vi "Autonomous Independent.vi"() -> ()   [LabVIEW 2012]
doc: "This VI is called when autonomous begins, and will automatically be terminated when autonomous ends. You can carry out timed or sensor driven robot movement independently without needing to return to the caller."
uses:
  <vilib>/Rock Robotics/WPI/Relay/WPI_RelayValue.ctl
  <vilib>/Rock Robotics/WPI/RobotDrive/WPI_RobotDriveGetSetRefNum.vi
  Robot Global Data.vi
panel:
  out "Shooter Up":bool
  out "Shooter Speed":T1(ring)
  out "Stop Drive":bool
  out "DT Output":enum16{"Off", "Up", "Down"}(ring)=enum."Down"
  out "DAD Up":bool
  out "DAD Output":T2
  out "Shift Low":bool
  out "Feeder Happy":bool
  out "Auton Done":bool
  out "Shooter Happy":bool
  out "Shoot!":bool
  out "Delay Switch":u32
  out "Seccond Switch":u32
  out "First Switch":u32
  # "Be sure to right-click and choose Data Operations>>Make Current Value default if you want to save the array values with the VI"
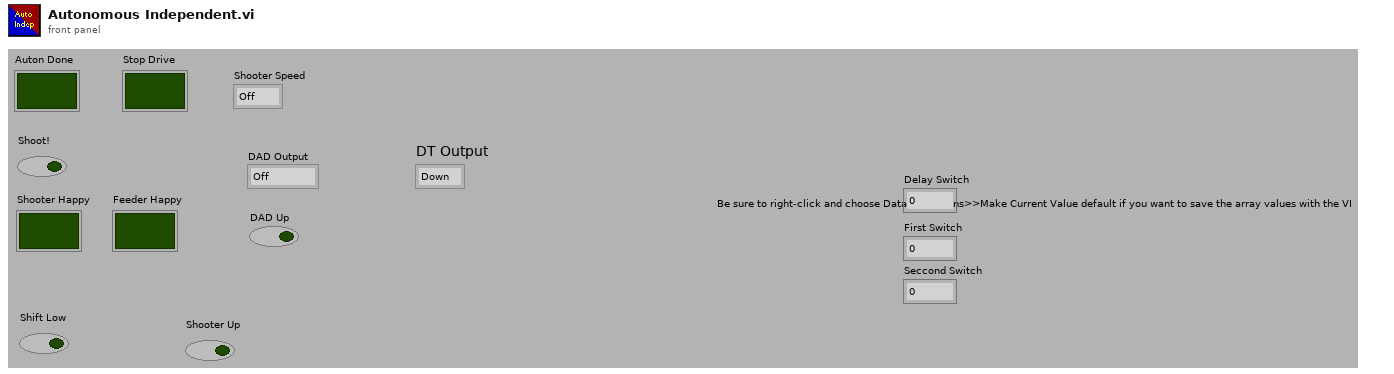
[diagram p1: front panel]
types:
  T1 = enum16{"Off", "Close Pyramid 3pt", "Far Pyramid 3pt", "Feeder Shot", "UD Far 3pt Shot"}
  T2 = typedef "WPI_RelayValue.ctl" = enum16{"Off", "On", "Forward", "Reverse"}
  T3 = enum16{"Off", "Close Pyramid 3pt", "Far Pyramid 3pt", "Feeder Shot"}
  T4 = typedef "WPI_RobotDriveDevRef.ctl" = cluster{"DevStatus":errorcluster, "Motors[]":T5[], "Square Inputs":bool, "Max Output":dbl, "Isochronous":bool}
  T5 = typedef "WPI_MotorControlDeviceRef.ctl" = cluster{"DeviceStatus":errorcluster, "Type":enum16{"PWM", "CAN"}, "PWM":cluster{"Digital Module":T6, "PWM Channel":T7, "DeadBand":T8}, "CAN":cluster{"Device Number":u8, "Control Mode":T9, "Semaphore":T10, "Max Vout":dbl}, "Invert":bool, "TransformRef":T11, "InvTransformRef":T11}
  T6 = typedef "FPGA_TypedefDigitalModule.ctl" = enum16{"Digital Module 1", "Digital Module 2"}
  T7 = typedef "FPGA_DIOPWMChannel.ctl" = enum8{"PWM 1", "PWM 2", "PWM 3", "PWM 4", "PWM 5", "PWM 6", "PWM 7", "PWM 8", "PWM 9", "PWM 10", "Invalid"}
  T8 = typedef "WPI_PWMDeadband.ctl" = cluster{"Name":string, "maxPositivePwm":i32, "minPositivePwm":i32, "centerPwm":i32, "maxNegativePwm":i32, "minNegativePwm":i32, "angularRange":u16}
  T9 = typedef "WPI_CANJaguar_ControlMode.ctl" = enum8{"Percent VBus", "Current", "Speed", "Position", "Voltage"}
  T10 = typedef "Semaphore RefNum" = refnum<k1>
  T11 = typedef "WPI_PWMTransform_ConPane.ctl" = refnum<vi>
  T12 = typedef "WPI_GyroDevRef.ctl" = cluster{"DevStatus":errorcluster, "Analog Module":T13, "Analog Channel":T14, "Offset":dbl, "Gain (VoltsPerDegree/Second)":dbl}
  T13 = typedef "FPGA_TypedefAnalogModule.ctl" = enum16{"Analog Module 1", "Analog Module 2"}
  T14 = typedef "FPGA_AIChannel.ctl" = enum8{"AI 1", "AI 2", "AI 3", "AI 4", "AI 5", "AI 6", "AI 7", "AI 8", "Invalid"}
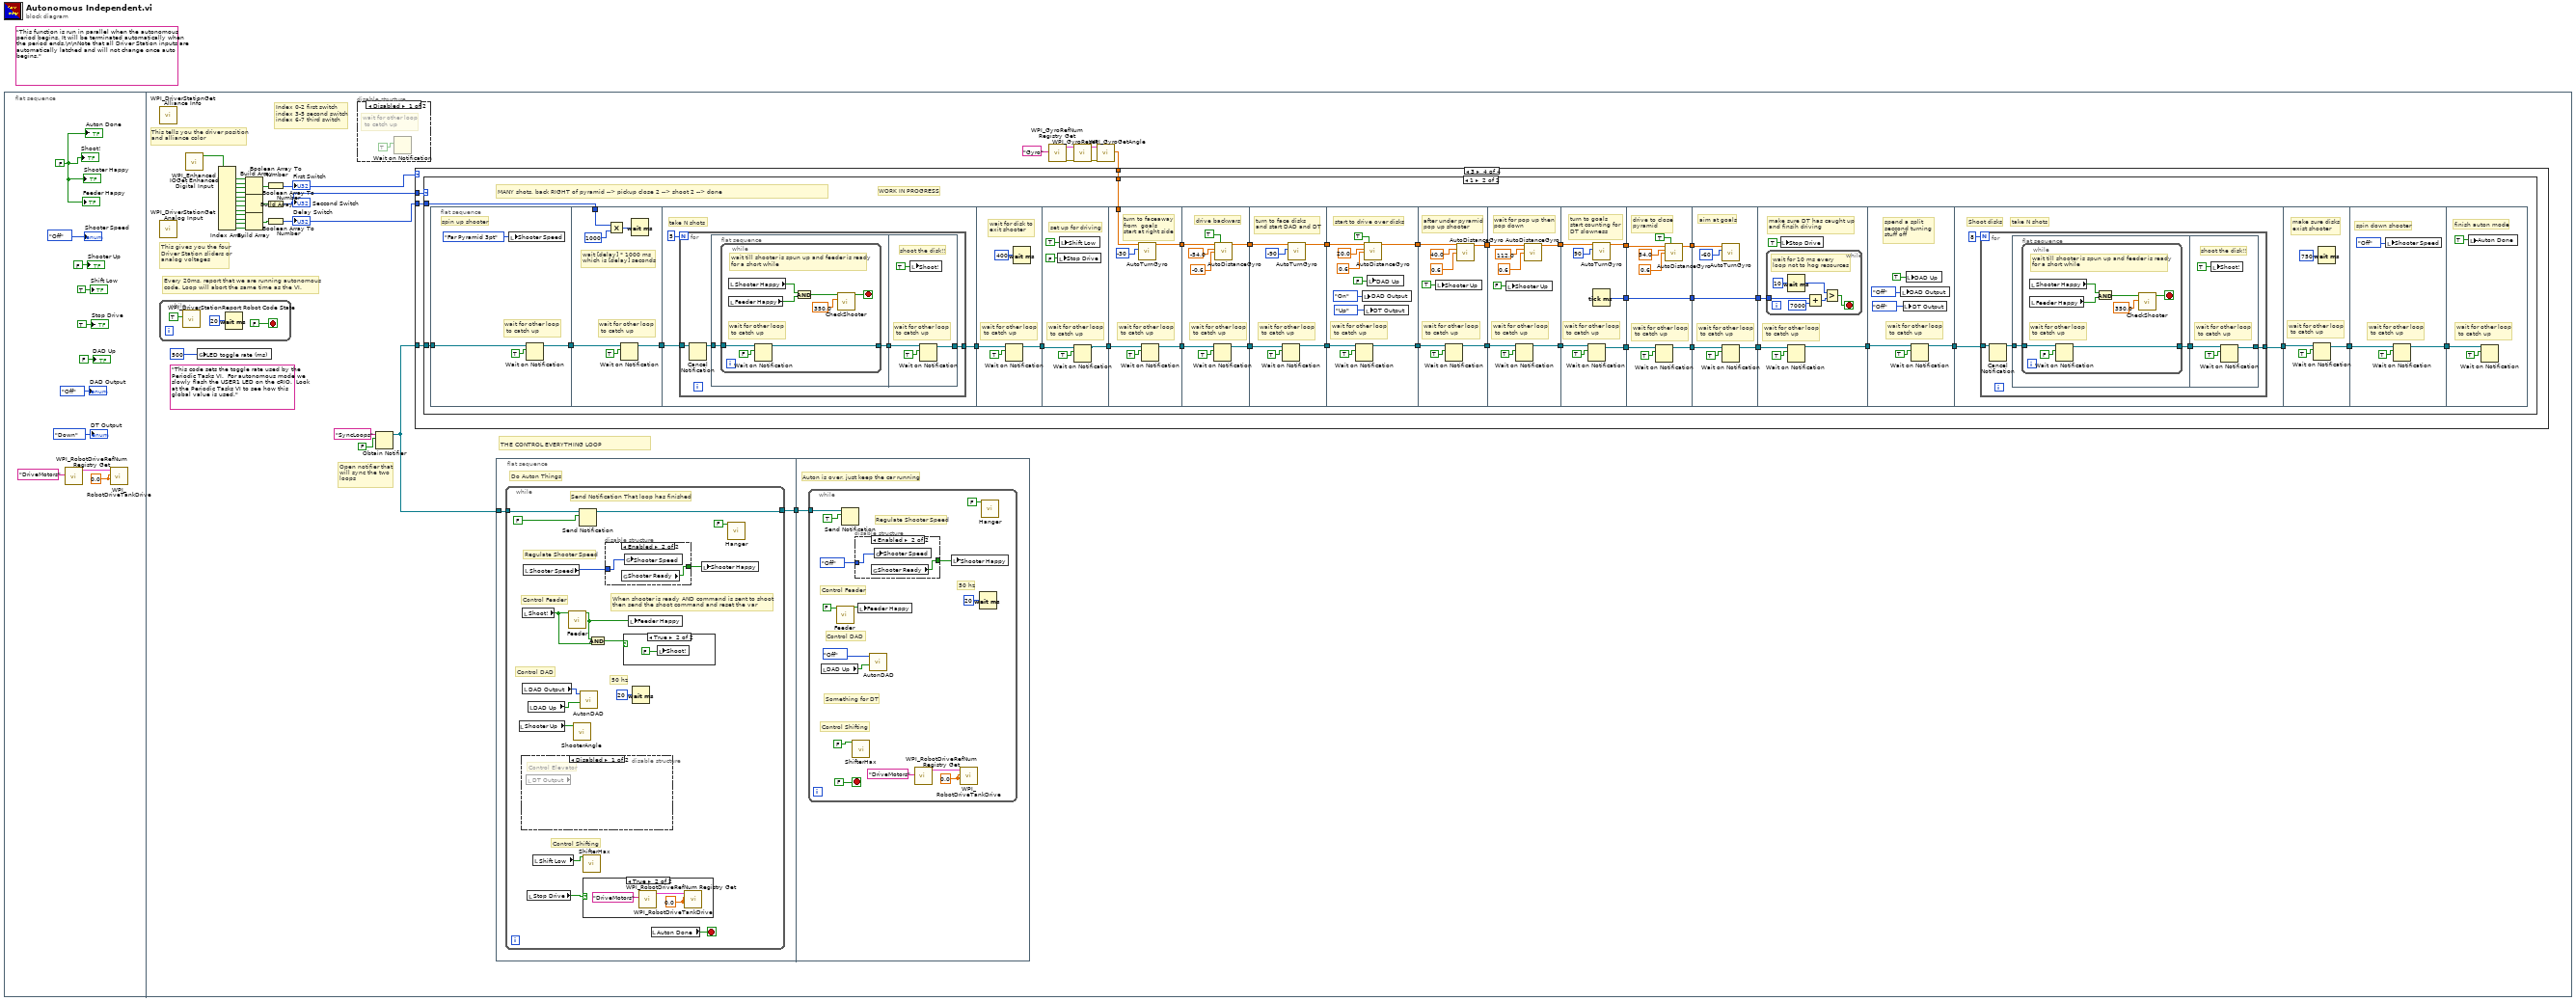
[diagram p0: block diagram]
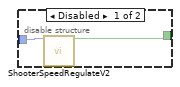
[diagram p3: hidden frame]
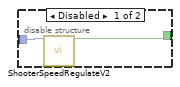
[diagram p7: hidden frame]
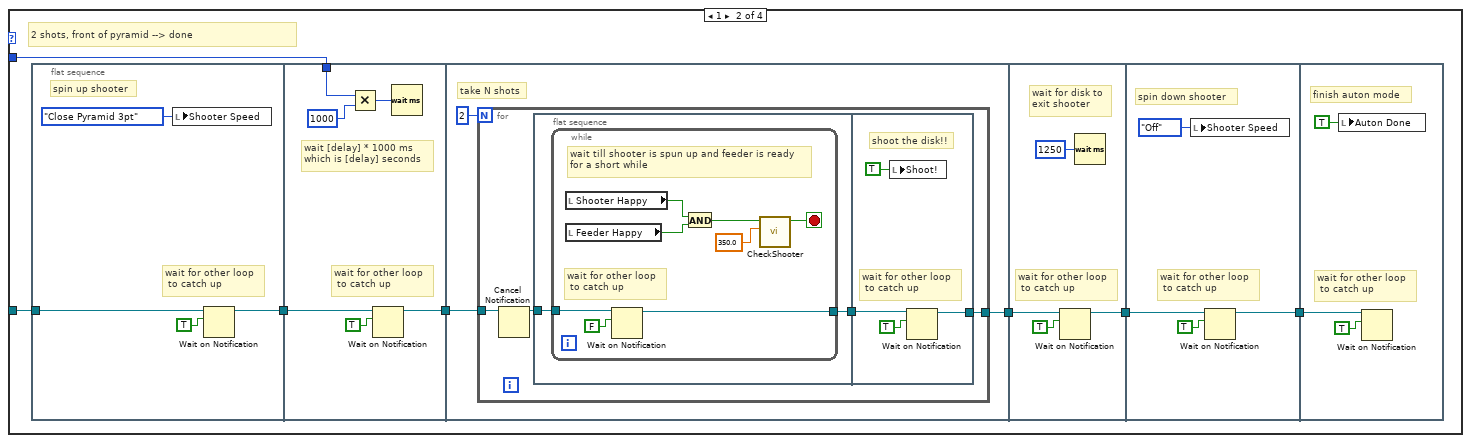
[diagram p10: hidden frame]
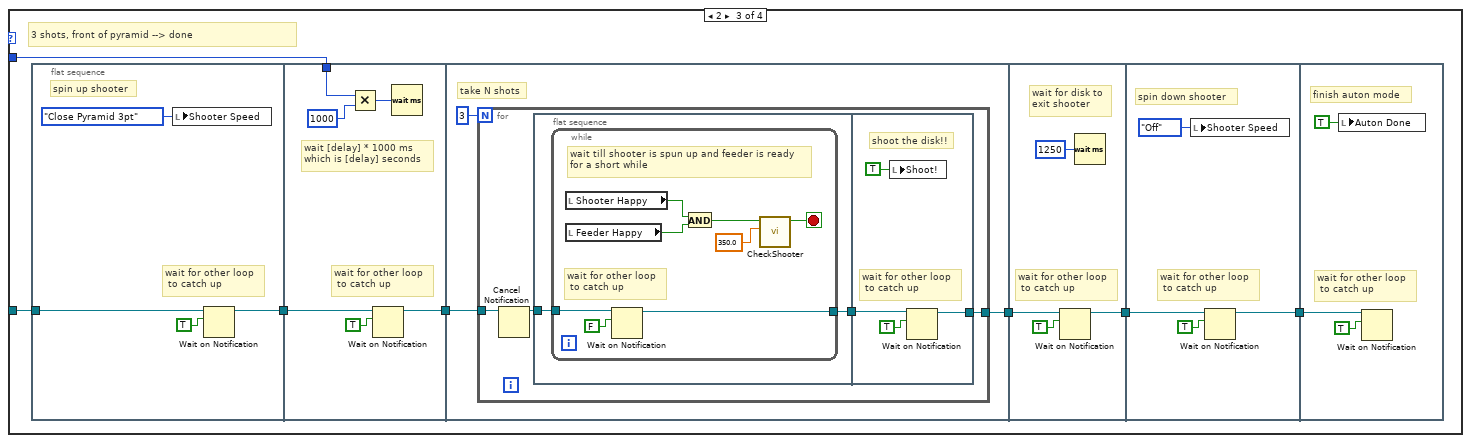
[diagram p11: hidden frame]
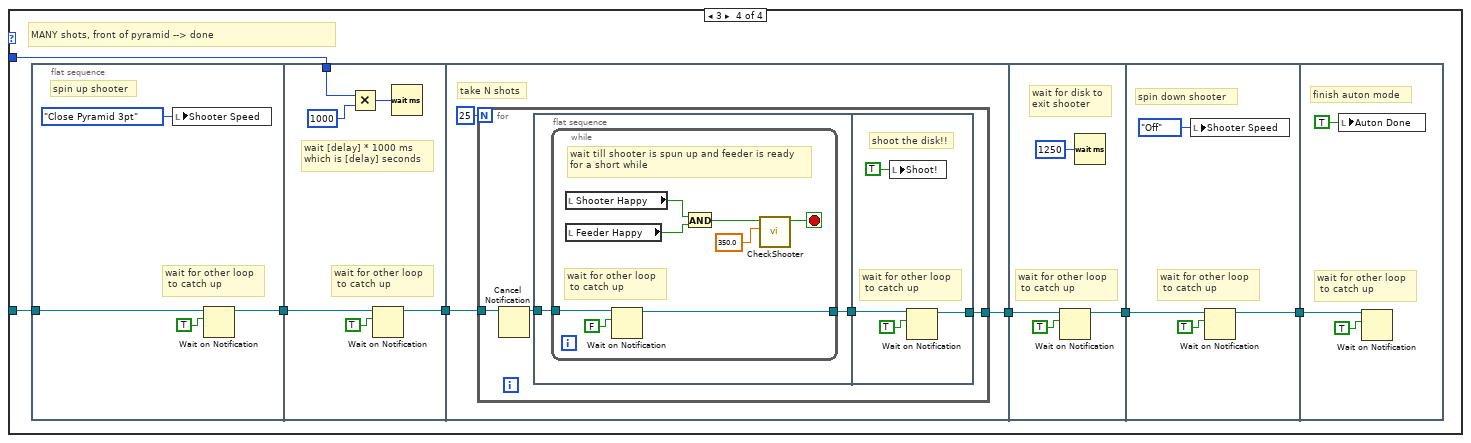
[diagram p12: hidden frame]
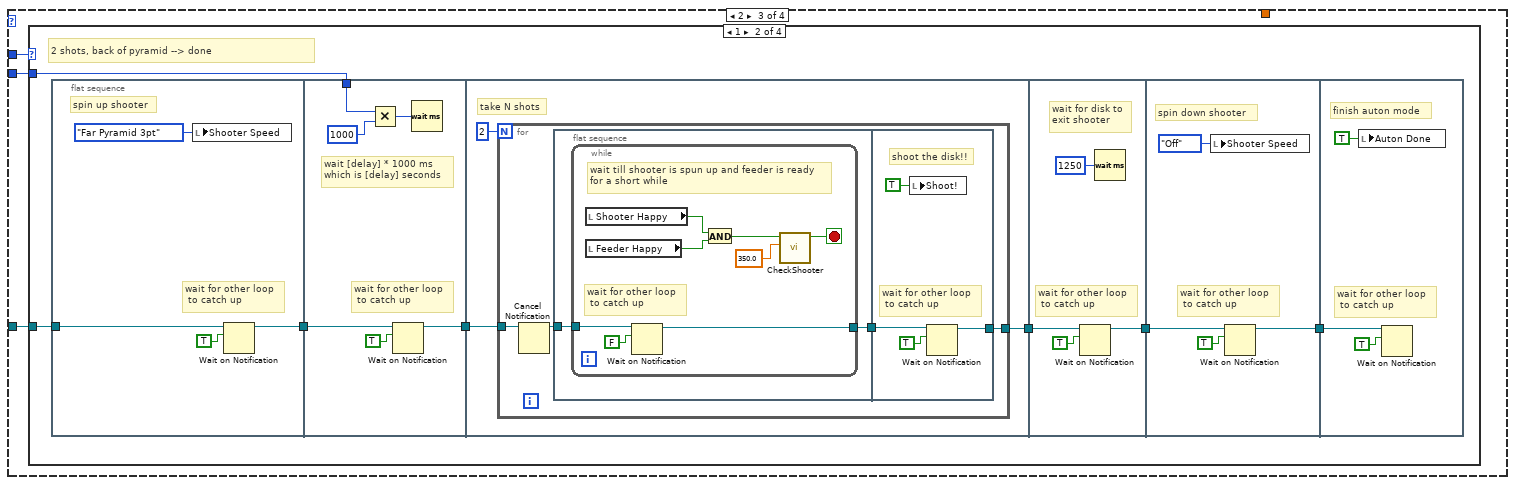
[diagram p13: hidden frame]
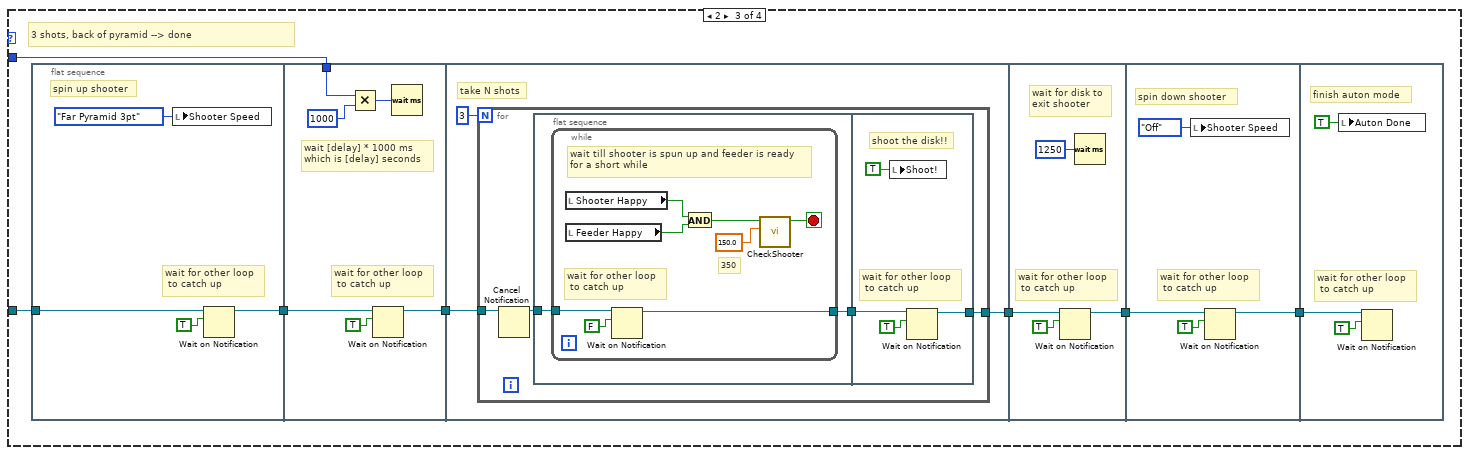
[diagram p15: hidden frame]
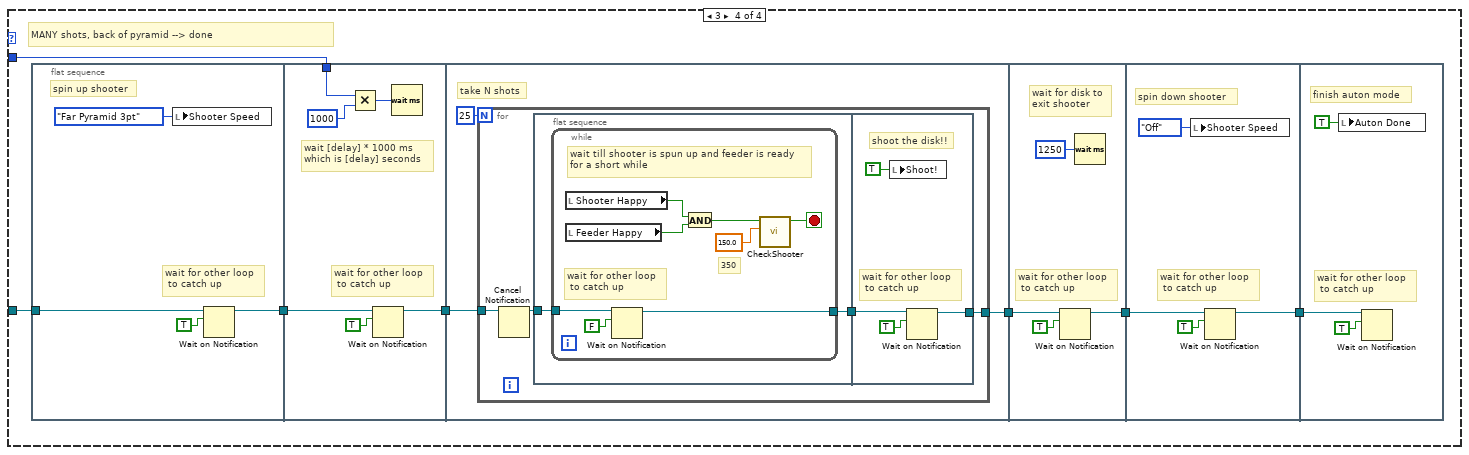
[diagram p16: hidden frame]
diagram:
  (unwired) "This function is run in parallel when the autonomous period begins. It will be terminated automatically when the period ends.\n\nNote that all Driver Station inputs are automatically latched and will not change once auto begins."
  n1 = flat-sequence {
    frame #0 {
      w4 = 0.0 ("Left axis value")
      w11 = FALSE
      n2 = call <vilib>:"WPI_RobotDriveRefNum Registry Get.vi"("refnum name"="DriveMotors") -> ("RobotDriveDevRef"=w6:T4)  [unwired: 1 in, 9 out]
      n3 = call <vilib>:"WPI_RobotDriveTankDrive.vi"("Right axis value"=w4, "Left axis value"=w4, "RobotDriveDevRef"=w6) -> ()  [unwired: 6 in, 3 out]
      "Feeder Happy" <- w11
      "Shift Low" <- TRUE ("Shift Low")
      "DAD Output" <- WPI_RelayValue."Off" ("DAD Output")
      "DAD Up" <- FALSE ("BAD Up")
      "Stop Drive" <- TRUE ("Stop Drive")
      "Shoot!" <- w11
      "Shooter Happy" <- w11
      "Auton Done" <- w11
      "DT Output" <- enum16{"Off", "Up", "Down"}."Down" ("DT Output")
      "Shooter Speed" <- T3."Off" ("Shooter Speed")
      "Shooter Up" <- FALSE ("Shooter Angle")
    }
    frame #1 {
      (unwired) "This code sets the toggle rate used by the Periodic Tasks VI.  For autonomous mode we slowly flash the USER1 LED on the cRIO.  Look at the Periodic Tasks VI to see how this global value is used."
      # "THE CONTROL EVERYTHING LOOP"
      # "Index 0-2 first switch\nindex 3-5 second switch\nindex 6-7 third switch"
      # "Open notifier that\nwill sync the two\nloops"
      # "Every 20ms, report that we are running autonomous\ncode. Loop will abort the same time as the VI."
      # "This tells you the driver position\nand alliance color"
      # "This gives you the four\nDriver Station sliders or\nanalog voltages"
      n4 = call <vilib>:"WPI_DriverStationGet Alliance Info.vi"() -> ()  [unwired: 12 out]
      n5 = call <vilib>:"WPI_DriverStationGet Analog Input.vi"() -> ()  [unwired: 12 out]
      n6 = while {
        stop <- FALSE stop-if-true
        n7 = call <vilib>:"WPI_DriverStationReport Robot Code State.vi"("Autonomous"=TRUE) -> ()  [unwired: 10 in, 1 out]
        n8 = Wait (ms)(milliseconds to wait=u32 20) -> ()  [unwired: 1 out]
      }
      n9 = call <vilib>:"WPI_Enhanced IOGet Enhanced Digital Input.vi"() -> ("Digital Input [1-16]"=w21:bool[])  [unwired: 10 in, 1 out]
      n10 = global write "Robot Global Data.vi" "LED toggle rate (ms)"(u32 500 ("LED ms toggle rate")) -> ()
      n11 = Index Array(array=w21) -> (element #1=w37:bool, element #2=w36:bool, element #3=w35:bool, element #4=w27:bool, element #5=w34:bool, element #6=w33:bool, element #7=w29:bool, element #8=w28:bool, element #9=w26:bool, element #10=w25:bool, element #11=w24:bool, element #12=w23:bool)  [unwired: 12 in]
      n12 = Build Array(w37, w36, w35, w27) -> (w31:bool[])
      n13 = Build Array(w34, w33, w29, w28) -> (w32:bool[])
      n14 = Build Array(w26, w25, w24, w23) -> (w22:bool[])
      n15 = Boolean Array To Number(Boolean array=w31) -> (number=w20:u32)
      "First Switch" <- w20
      n16 = Boolean Array To Number(Boolean array=w32) -> (number=w19:u32)
      "Seccond Switch" <- w19
      n17 = Boolean Array To Number(Boolean array=w22) -> (number=w17:u32)
      "Delay Switch" <- w17
      n18 = disable-structure shown="Disabled" {
        frame Disabled {
          # "wait for other loop\n to catch up"
          n19 = Wait on Notification(ignore previous (F)=TRUE) -> (notifier=w43:refnum<notifier>)  [unwired: 2 in, 4 out]
        }
        frame Enabled {
        }
      }
      n20 = Obtain Notifier(name (unnamed)="SyncLoops", notification data type=FALSE) -> (notifier out=w18:refnum<notifier>)  [unwired: 2 in, 2 out]
      n21 = flat-sequence {
        tunnel: w18 -> [w45]
        tunnel: [w44] -> w41
        tunnel: w41 -> [w70]
        frame #0 {
          # "Do Auton Things"
          n22 = while {
            tunnel: w45 -> [w59]
            tunnel: [w55] -> w44
            stop <- w61 stop-if-true
            # "Regulate Shooter Speed"
            # "50 hz"
            # "Control DAD"
            # "Control Shifting"
            # "When shooter is ready AND command is sent to shoot\nthen send the shoot command and reset the var"
            # "Control Feader"
            # "Send Notification That loop has finished"
            n23 = local read "Shooter Up"() -> (w46:bool)
            n24 = disable-structure shown="Disabled" {
              frame Disabled {
                # "Control Elevator"
                n25 = local read "DT Output"() -> ()  [unwired: 1 out]
              }
              frame Enabled {
              }
            }
            n26 = local read "Shoot!"() -> (w58:bool)
            n27 = local read "DAD Output"() -> (w51:T2)
            n28 = local read "Shooter Speed"() -> (w48:T1)
            n29 = local read "Stop Drive"() -> (w53:bool)
            n30 = local read "DAD Up"() -> (w52:bool)
            n31 = local read "Shift Low"() -> (w49:bool)
            n32 = call "Feeder.vi"("SHOOT Button"=w58) -> ("Ready To Shoot?"=w56:bool)  [unwired: 10 in]
            n33 = call "ShooterAngle.vi"("Shooter Angle Up?"=w46) -> ()  [unwired: 10 in, 1 out]
            n34 = Send Notification(notification=FALSE, notifier=w59) -> (notifier out=w55:refnum<notifier>)  [unwired: 1 in, 1 out]
            n35 = call "AutonDAD.vi"("BAD UP"=w52, "BAD Output"=w51) -> ()  [unwired: 10 in]
            n36 = case shown="True" w53 {
              frame False {
              }
              frame True {
                w68 = 0.0 ("Left axis value")
                n37 = call <vilib>:"WPI_RobotDriveRefNum Registry Get.vi"("refnum name"="DriveMotors") -> ("RobotDriveDevRef"=w66:T4)  [unwired: 1 in, 9 out]
                n38 = call <vilib>:"WPI_RobotDriveTankDrive.vi"("Right axis value"=w68, "Left axis value"=w68, "RobotDriveDevRef"=w66) -> ()  [unwired: 6 in, 3 out]
              }
            }
            n39 = call "ShifterHax.vi"("Shift low?"=w49) -> ()  [unwired: 11 in]
            n40 = And(x=w56, y=w58) -> (x .and. y?=w57:bool)
            n41 = disable-structure shown="Enabled" {
              disable-tunnel: [w63 w64] -> w50
              disable-tunnel: w48 -> [w62 w65]
              frame Disabled {
                n42 = call "ShooterSpeedRegulateV2.vi"("Shooter Speed"=w62) -> ("ALL GOOD"=w63:bool)  [unwired: 13 in, 1 out]
              }
              frame Enabled {
                n43 = global read "Robot Global Data.vi" "Shooter Ready"() -> (w64:bool)
                n44 = global write "Robot Global Data.vi" "Shooter Speed"(w65) -> ()
              }
            }
            n45 = case shown="True" w57 {
              frame False {
              }
              frame True {
                n46 = local write "Shoot!"(FALSE) -> ()
              }
            }
            n47 = local write "Feeder Happy"(w56) -> ()
            n48 = Wait (ms)(milliseconds to wait=u32 20) -> ()  [unwired: 1 out]
            n49 = local read "Auton Done"() -> (w61:bool)
            n50 = local write "Shooter Happy"(w50) -> ()
            n51 = call "Hanger.vi"("Hanger Up"=FALSE) -> ()  [unwired: 10 in, 1 out]
          }
        }
        frame #1 {
          # "Auton is over, just keep the car running"
          n52 = while {
            tunnel: w70 -> [w75]
            stop <- FALSE stop-if-true
            w80 = 0.0 ("Left axis value")
            # "Something for DT"
            # "50 hz"
            # "Regulate Shooter Speed"
            # "Control DAD"
            # "Control Shifting"
            # "Control Feader"
            n53 = local read "DAD Up"() -> (w78:bool)
            n54 = call "Feeder.vi"("SHOOT Button"=FALSE) -> ("Ready To Shoot?"=w84:bool)  [unwired: 10 in]
            n55 = Send Notification(notification=TRUE, notifier=w75) -> ()  [unwired: 1 in, 2 out]
            n56 = call "ShifterHax.vi"("Shift low?"=FALSE ("Shifting Button")) -> ()  [unwired: 11 in]
            n57 = disable-structure shown="Enabled" {
              disable-tunnel: [w87 w88] -> w72
              disable-tunnel: T3."Off" ("Shooter Speed") -> [w86 w89]
              frame Disabled {
                n58 = call "ShooterSpeedRegulateV2.vi"("Shooter Speed"=w86) -> ("ALL GOOD"=w87:bool)  [unwired: 13 in, 1 out]
              }
              frame Enabled {
                n59 = global read "Robot Global Data.vi" "Shooter Ready"() -> (w88:bool)
                n60 = global write "Robot Global Data.vi" "Shooter Speed"(w89) -> ()
              }
            }
            n61 = local write "Feeder Happy"(w84) -> ()
            n62 = call "AutonDAD.vi"("BAD UP"=w78, "BAD Output"=WPI_RelayValue."Off") -> ()  [unwired: 10 in]
            n63 = call <vilib>:"WPI_RobotDriveRefNum Registry Get.vi"("refnum name"="DriveMotors") -> ("RobotDriveDevRef"=w82:T4)  [unwired: 1 in, 9 out]
            n64 = local write "Shooter Happy"(w72) -> ()
            n65 = call <vilib>:"WPI_RobotDriveTankDrive.vi"("Right axis value"=w80, "Left axis value"=w80, "RobotDriveDevRef"=w82) -> ()  [unwired: 6 in, 3 out]
            n66 = Wait (ms)(milliseconds to wait=u32 20) -> ()  [unwired: 1 out]
            n67 = call "Hanger.vi"("Hanger Up"=FALSE) -> ()  [unwired: 10 in, 1 out]
          }
        }
      }
      n68 = call <vilib>:"WPI_GyroRefNum Registry Get.vi"("refnum name"="Gyro") -> ("error out"=w16:errorcluster, "GyroDevRef"=w15:T12)  [unwired: 9 in]
      n69 = call <vilib>:"WPI_GyroReset.vi"("error in (no error)"=w16, "GyroDevRef"=w15) -> ("error out"=w14:errorcluster, "GyroDevRef"=w13:T12)  [unwired: 8 in]
      n70 = call <vilib>:"WPI_GyroGetAngle.vi"("error in (no error)"=w14, "GyroDevRef"=w13) -> ("Angle"=w12:dbl)  [unwired: 6 in, 3 out]
      n71 = case shown="3" w20 {
        tunnel: w19 -> [_ w92 w242 w393]
        tunnel: w18 -> [_ w91 w241 w392]
        tunnel: w17 -> [_ w90 w240 w391]
        tunnel: w12 -> [_ _ _ w390]
        frame 0, Default {
          # "do nothing"
        }
        frame 1 {
          n72 = case shown="0, Default" w92 {
            tunnel: w91 -> [_ w96 w145 w194]
            tunnel: w90 -> [_ w99 w148 w197]
            frame 0, Default {
              # "do nothing"
            }
            frame 1 {
              # "2 shots, front of pyramid --> done"
              n73 = flat-sequence {
                tunnel: [w102] -> w98
                tunnel: w96 -> [w101]
                tunnel: w99 -> [w107]
                tunnel: w98 -> [w105]
                tunnel: [w104] -> w97
                tunnel: w97 -> [w111]
                tunnel: [w110] -> w93
                tunnel: [w132] -> w94
                tunnel: w93 -> [w131]
                tunnel: [w137] -> w95
                tunnel: w94 -> [w136]
                tunnel: w95 -> [w139]
                frame #0 {
                  # "wait for other loop\n to catch up"
                  # "spin up shooter"
                  n74 = local write "Shooter Speed"(T3."Close Pyramid 3pt" ("Shooter Speed")) -> ()
                  n75 = Wait on Notification(notifier=w101, ignore previous (F)=TRUE) -> (notifier out=w102:refnum<notifier>)  [unwired: 2 in, 3 out]
                }
                frame #1 {
                  # "wait for other loop\n to catch up"
                  # "wait [delay] * 1000 ms\nwhich is [delay] seconds"
                  n76 = Multiply(x=w107, y=1000) -> (x*y=w109:u32)
                  n77 = Wait on Notification(notifier=w105, ignore previous (F)=TRUE) -> (notifier out=w104:refnum<notifier>)  [unwired: 2 in, 3 out]
                  n78 = Wait (ms)(milliseconds to wait=w109) -> ()  [unwired: 1 out]
                }
                frame #2 {
                  # "take N shots"
                  n79 = for {
                    N: 2 -> [_]
                    tunnel: w111 -> [w115]
                    tunnel: [w113] -> w110
                    n80 = Cancel Notification(0:w115) -> (8:w116:refnum<notifier>)  [unwired: 1 in, 2 out]
                    n81 = flat-sequence {
                      tunnel: w116 -> [w118]
                      tunnel: [w117] -> w114
                      tunnel: w114 -> [w128]
                      tunnel: [w127] -> w113
                      frame #0 {
                        n82 = while {
                          tunnel: w118 -> [w120]
                          tunnel: [w119] -> w117
                          stop <- w122 stop-if-true
                          # "wait for other loop\n to catch up"
                          # "wait till shooter is spun up and feeder is ready\nfor a short while"
                          n83 = local read "Shooter Happy"() -> (w125:bool)
                          n84 = local read "Feeder Happy"() -> (w124:bool)
                          n85 = Wait on Notification(notifier=w120, ignore previous (F)=FALSE) -> (notifier out=w119:refnum<notifier>)  [unwired: 2 in, 3 out]
                          n86 = And(x=w125, y=w124) -> (x .and. y?=w123:bool)
                          n87 = call "CheckShooter.vi"("Time for happy (ms)"=350.0, "Shooter Good?"=w123) -> ("Good to shoot"=w122:bool)  [unwired: 9 in]
                        }
                      }
                      frame #1 {
                        # "wait for other loop\n to catch up"
                        # "shoot the disk!!"
                        n88 = local write "Shoot!"(TRUE ("Shoot!")) -> ()
                        n89 = Wait on Notification(notifier=w128, ignore previous (F)=TRUE) -> (notifier out=w127:refnum<notifier>)  [unwired: 2 in, 3 out]
                      }
                    }
                  }
                }
                frame #3 {
                  # "wait for other loop\n to catch up"
                  # "wait for disk to\nexit shooter"
                  n90 = Wait on Notification(notifier=w131, ignore previous (F)=TRUE) -> (notifier out=w132:refnum<notifier>)  [unwired: 2 in, 3 out]
                  n91 = Wait (ms)(milliseconds to wait=u32 1250) -> ()  [unwired: 1 out]
                }
                frame #4 {
                  # "wait for other loop\n to catch up"
                  # "spin down shooter"
                  n92 = local write "Shooter Speed"(T3."Off" ("Shooter Speed")) -> ()
                  n93 = Wait on Notification(notifier=w136, ignore previous (F)=TRUE) -> (notifier out=w137:refnum<notifier>)  [unwired: 2 in, 3 out]
                }
                frame #5 {
                  # "wait for other loop\n to catch up"
                  # "finish auton mode"
                  n94 = local write "Auton Done"(TRUE ("Auton Done")) -> ()
                  n95 = Wait on Notification(notifier=w139, ignore previous (F)=TRUE) -> ()  [unwired: 2 in, 4 out]
                }
              }
            }
            frame 2 {
              # "3 shots, front of pyramid --> done"
              n96 = flat-sequence {
                tunnel: [w151] -> w147
                tunnel: w145 -> [w150]
                tunnel: w148 -> [w156]
                tunnel: w147 -> [w154]
                tunnel: [w153] -> w146
                tunnel: w146 -> [w160]
                tunnel: [w159] -> w142
                tunnel: [w181] -> w143
                tunnel: w142 -> [w180]
                tunnel: [w186] -> w144
                tunnel: w143 -> [w185]
                tunnel: w144 -> [w188]
                frame #0 {
                  # "wait for other loop\n to catch up"
                  # "spin up shooter"
                  n97 = local write "Shooter Speed"(T3."Close Pyramid 3pt" ("Shooter Speed")) -> ()
                  n98 = Wait on Notification(notifier=w150, ignore previous (F)=TRUE) -> (notifier out=w151:refnum<notifier>)  [unwired: 2 in, 3 out]
                }
                frame #1 {
                  # "wait for other loop\n to catch up"
                  # "wait [delay] * 1000 ms\nwhich is [delay] seconds"
                  n99 = Multiply(x=w156, y=1000) -> (x*y=w158:u32)
                  n100 = Wait on Notification(notifier=w154, ignore previous (F)=TRUE) -> (notifier out=w153:refnum<notifier>)  [unwired: 2 in, 3 out]
                  n101 = Wait (ms)(milliseconds to wait=w158) -> ()  [unwired: 1 out]
                }
                frame #2 {
                  # "take N shots"
                  n102 = for {
                    N: 3 -> [_]
                    tunnel: w160 -> [w164]
                    tunnel: [w162] -> w159
                    n103 = Cancel Notification(0:w164) -> (8:w165:refnum<notifier>)  [unwired: 1 in, 2 out]
                    n104 = flat-sequence {
                      tunnel: w165 -> [w167]
                      tunnel: [w166] -> w163
                      tunnel: w163 -> [w177]
                      tunnel: [w176] -> w162
                      frame #0 {
                        n105 = while {
                          tunnel: w167 -> [w169]
                          tunnel: [w168] -> w166
                          stop <- w171 stop-if-true
                          # "wait for other loop\n to catch up"
                          # "wait till shooter is spun up and feeder is ready\nfor a short while"
                          n106 = local read "Shooter Happy"() -> (w174:bool)
                          n107 = local read "Feeder Happy"() -> (w173:bool)
                          n108 = Wait on Notification(notifier=w169, ignore previous (F)=FALSE) -> (notifier out=w168:refnum<notifier>)  [unwired: 2 in, 3 out]
                          n109 = And(x=w174, y=w173) -> (x .and. y?=w172:bool)
                          n110 = call "CheckShooter.vi"("Time for happy (ms)"=350.0, "Shooter Good?"=w172) -> ("Good to shoot"=w171:bool)  [unwired: 9 in]
                        }
                      }
                      frame #1 {
                        # "wait for other loop\n to catch up"
                        # "shoot the disk!!"
                        n111 = local write "Shoot!"(TRUE ("Shoot!")) -> ()
                        n112 = Wait on Notification(notifier=w177, ignore previous (F)=TRUE) -> (notifier out=w176:refnum<notifier>)  [unwired: 2 in, 3 out]
                      }
                    }
                  }
                }
                frame #3 {
                  # "wait for other loop\n to catch up"
                  # "wait for disk to\nexit shooter"
                  n113 = Wait on Notification(notifier=w180, ignore previous (F)=TRUE) -> (notifier out=w181:refnum<notifier>)  [unwired: 2 in, 3 out]
                  n114 = Wait (ms)(milliseconds to wait=u32 1250) -> ()  [unwired: 1 out]
                }
                frame #4 {
                  # "wait for other loop\n to catch up"
                  # "spin down shooter"
                  n115 = local write "Shooter Speed"(T3."Off" ("Shooter Speed")) -> ()
                  n116 = Wait on Notification(notifier=w185, ignore previous (F)=TRUE) -> (notifier out=w186:refnum<notifier>)  [unwired: 2 in, 3 out]
                }
                frame #5 {
                  # "wait for other loop\n to catch up"
                  # "finish auton mode"
                  n117 = local write "Auton Done"(TRUE ("Auton Done")) -> ()
                  n118 = Wait on Notification(notifier=w188, ignore previous (F)=TRUE) -> ()  [unwired: 2 in, 4 out]
                }
              }
            }
            frame 3 {
              # "MANY shots, front of pyramid --> done"
              n119 = flat-sequence {
                tunnel: [w200] -> w196
                tunnel: w194 -> [w199]
                tunnel: w197 -> [w205]
                tunnel: w196 -> [w203]
                tunnel: [w202] -> w195
                tunnel: w195 -> [w209]
                tunnel: [w208] -> w191
                tunnel: [w230] -> w192
                tunnel: w191 -> [w229]
                tunnel: [w235] -> w193
                tunnel: w192 -> [w234]
                tunnel: w193 -> [w237]
                frame #0 {
                  # "wait for other loop\n to catch up"
                  # "spin up shooter"
                  n120 = local write "Shooter Speed"(T3."Close Pyramid 3pt" ("Shooter Speed")) -> ()
                  n121 = Wait on Notification(notifier=w199, ignore previous (F)=TRUE) -> (notifier out=w200:refnum<notifier>)  [unwired: 2 in, 3 out]
                }
                frame #1 {
                  # "wait for other loop\n to catch up"
                  # "wait [delay] * 1000 ms\nwhich is [delay] seconds"
                  n122 = Multiply(x=w205, y=1000) -> (x*y=w207:u32)
                  n123 = Wait on Notification(notifier=w203, ignore previous (F)=TRUE) -> (notifier out=w202:refnum<notifier>)  [unwired: 2 in, 3 out]
                  n124 = Wait (ms)(milliseconds to wait=w207) -> ()  [unwired: 1 out]
                }
                frame #2 {
                  # "take N shots"
                  n125 = for {
                    N: 25 -> [_]
                    tunnel: w209 -> [w213]
                    tunnel: [w211] -> w208
                    n126 = Cancel Notification(0:w213) -> (8:w214:refnum<notifier>)  [unwired: 1 in, 2 out]
                    n127 = flat-sequence {
                      tunnel: w214 -> [w216]
                      tunnel: [w215] -> w212
                      tunnel: w212 -> [w226]
                      tunnel: [w225] -> w211
                      frame #0 {
                        n128 = while {
                          tunnel: w216 -> [w218]
                          tunnel: [w217] -> w215
                          stop <- w220 stop-if-true
                          # "wait for other loop\n to catch up"
                          # "wait till shooter is spun up and feeder is ready\nfor a short while"
                          n129 = local read "Shooter Happy"() -> (w223:bool)
                          n130 = local read "Feeder Happy"() -> (w222:bool)
                          n131 = Wait on Notification(notifier=w218, ignore previous (F)=FALSE) -> (notifier out=w217:refnum<notifier>)  [unwired: 2 in, 3 out]
                          n132 = And(x=w223, y=w222) -> (x .and. y?=w221:bool)
                          n133 = call "CheckShooter.vi"("Time for happy (ms)"=350.0, "Shooter Good?"=w221) -> ("Good to shoot"=w220:bool)  [unwired: 9 in]
                        }
                      }
                      frame #1 {
                        # "wait for other loop\n to catch up"
                        # "shoot the disk!!"
                        n134 = local write "Shoot!"(TRUE ("Shoot!")) -> ()
                        n135 = Wait on Notification(notifier=w226, ignore previous (F)=TRUE) -> (notifier out=w225:refnum<notifier>)  [unwired: 2 in, 3 out]
                      }
                    }
                  }
                }
                frame #3 {
                  # "wait for other loop\n to catch up"
                  # "wait for disk to\nexit shooter"
                  n136 = Wait on Notification(notifier=w229, ignore previous (F)=TRUE) -> (notifier out=w230:refnum<notifier>)  [unwired: 2 in, 3 out]
                  n137 = Wait (ms)(milliseconds to wait=u32 1250) -> ()  [unwired: 1 out]
                }
                frame #4 {
                  # "wait for other loop\n to catch up"
                  # "spin down shooter"
                  n138 = local write "Shooter Speed"(T3."Off" ("Shooter Speed")) -> ()
                  n139 = Wait on Notification(notifier=w234, ignore previous (F)=TRUE) -> (notifier out=w235:refnum<notifier>)  [unwired: 2 in, 3 out]
                }
                frame #5 {
                  # "wait for other loop\n to catch up"
                  # "finish auton mode"
                  n140 = local write "Auton Done"(TRUE ("Auton Done")) -> ()
                  n141 = Wait on Notification(notifier=w237, ignore previous (F)=TRUE) -> ()  [unwired: 2 in, 4 out]
                }
              }
            }
          }
        }
        frame 2 {
          n142 = case shown="1" w242 {
            tunnel: w241 -> [_ w246 w295 w344]
            tunnel: w240 -> [_ w249 w298 w347]
            frame 0, Default {
              # "do nothing"
            }
            frame 1 {
              # "2 shots, back of pyramid --> done"
              n143 = flat-sequence {
                tunnel: [w252] -> w248
                tunnel: w246 -> [w251]
                tunnel: w249 -> [w257]
                tunnel: w248 -> [w255]
                tunnel: [w254] -> w247
                tunnel: w247 -> [w261]
                tunnel: [w260] -> w243
                tunnel: [w282] -> w244
                tunnel: w243 -> [w281]
                tunnel: [w287] -> w245
                tunnel: w244 -> [w286]
                tunnel: w245 -> [w289]
                frame #0 {
                  # "wait for other loop\n to catch up"
                  # "spin up shooter"
                  n144 = local write "Shooter Speed"(T3."Far Pyramid 3pt" ("Shooter Speed")) -> ()
                  n145 = Wait on Notification(notifier=w251, ignore previous (F)=TRUE) -> (notifier out=w252:refnum<notifier>)  [unwired: 2 in, 3 out]
                }
                frame #1 {
                  # "wait for other loop\n to catch up"
                  # "wait [delay] * 1000 ms\nwhich is [delay] seconds"
                  n146 = Multiply(x=w257, y=1000) -> (x*y=w259:u32)
                  n147 = Wait on Notification(notifier=w255, ignore previous (F)=TRUE) -> (notifier out=w254:refnum<notifier>)  [unwired: 2 in, 3 out]
                  n148 = Wait (ms)(milliseconds to wait=w259) -> ()  [unwired: 1 out]
                }
                frame #2 {
                  # "take N shots"
                  n149 = for {
                    N: 2 -> [_]
                    tunnel: w261 -> [w265]
                    tunnel: [w263] -> w260
                    n150 = Cancel Notification(0:w265) -> (8:w266:refnum<notifier>)  [unwired: 1 in, 2 out]
                    n151 = flat-sequence {
                      tunnel: w266 -> [w268]
                      tunnel: [w267] -> w264
                      tunnel: w264 -> [w278]
                      tunnel: [w277] -> w263
                      frame #0 {
                        n152 = while {
                          tunnel: w268 -> [w270]
                          tunnel: [w269] -> w267
                          stop <- w272 stop-if-true
                          # "wait for other loop\n to catch up"
                          # "wait till shooter is spun up and feeder is ready\nfor a short while"
                          n153 = local read "Shooter Happy"() -> (w275:bool)
                          n154 = local read "Feeder Happy"() -> (w274:bool)
                          n155 = Wait on Notification(notifier=w270, ignore previous (F)=FALSE) -> (notifier out=w269:refnum<notifier>)  [unwired: 2 in, 3 out]
                          n156 = And(x=w275, y=w274) -> (x .and. y?=w273:bool)
                          n157 = call "CheckShooter.vi"("Time for happy (ms)"=350.0, "Shooter Good?"=w273) -> ("Good to shoot"=w272:bool)  [unwired: 9 in]
                        }
                      }
                      frame #1 {
                        # "wait for other loop\n to catch up"
                        # "shoot the disk!!"
                        n158 = local write "Shoot!"(TRUE ("Shoot!")) -> ()
                        n159 = Wait on Notification(notifier=w278, ignore previous (F)=TRUE) -> (notifier out=w277:refnum<notifier>)  [unwired: 2 in, 3 out]
                      }
                    }
                  }
                }
                frame #3 {
                  # "wait for other loop\n to catch up"
                  # "wait for disk to\nexit shooter"
                  n160 = Wait on Notification(notifier=w281, ignore previous (F)=TRUE) -> (notifier out=w282:refnum<notifier>)  [unwired: 2 in, 3 out]
                  n161 = Wait (ms)(milliseconds to wait=u32 1250) -> ()  [unwired: 1 out]
                }
                frame #4 {
                  # "wait for other loop\n to catch up"
                  # "spin down shooter"
                  n162 = local write "Shooter Speed"(T3."Off" ("Shooter Speed")) -> ()
                  n163 = Wait on Notification(notifier=w286, ignore previous (F)=TRUE) -> (notifier out=w287:refnum<notifier>)  [unwired: 2 in, 3 out]
                }
                frame #5 {
                  # "wait for other loop\n to catch up"
                  # "finish auton mode"
                  n164 = local write "Auton Done"(TRUE ("Auton Done")) -> ()
                  n165 = Wait on Notification(notifier=w289, ignore previous (F)=TRUE) -> ()  [unwired: 2 in, 4 out]
                }
              }
            }
            frame 2 {
              # "3 shots, back of pyramid --> done"
              n166 = flat-sequence {
                tunnel: [w301] -> w297
                tunnel: w295 -> [w300]
                tunnel: w298 -> [w306]
                tunnel: w297 -> [w304]
                tunnel: [w303] -> w296
                tunnel: w296 -> [w310]
                tunnel: [w309] -> w292
                tunnel: [w331] -> w293
                tunnel: w292 -> [w330]
                tunnel: [w336] -> w294
                tunnel: w293 -> [w335]
                tunnel: w294 -> [w338]
                frame #0 {
                  # "wait for other loop\n to catch up"
                  # "spin up shooter"
                  n167 = local write "Shooter Speed"(T3."Far Pyramid 3pt" ("Shooter Speed")) -> ()
                  n168 = Wait on Notification(notifier=w300, ignore previous (F)=TRUE) -> (notifier out=w301:refnum<notifier>)  [unwired: 2 in, 3 out]
                }
                frame #1 {
                  # "wait for other loop\n to catch up"
                  # "wait [delay] * 1000 ms\nwhich is [delay] seconds"
                  n169 = Multiply(x=w306, y=1000) -> (x*y=w308:u32)
                  n170 = Wait on Notification(notifier=w304, ignore previous (F)=TRUE) -> (notifier out=w303:refnum<notifier>)  [unwired: 2 in, 3 out]
                  n171 = Wait (ms)(milliseconds to wait=w308) -> ()  [unwired: 1 out]
                }
                frame #2 {
                  # "take N shots"
                  n172 = for {
                    N: 3 -> [_]
                    tunnel: w310 -> [w314]
                    tunnel: [w312] -> w309
                    n173 = Cancel Notification(0:w314) -> (8:w315:refnum<notifier>)  [unwired: 1 in, 2 out]
                    n174 = flat-sequence {
                      tunnel: w315 -> [w317]
                      tunnel: [w316] -> w313
                      tunnel: w313 -> [w327]
                      tunnel: [w326] -> w312
                      frame #0 {
                        n175 = while {
                          tunnel: w317 -> [w319]
                          tunnel: [w318] -> w316
                          stop <- w321 stop-if-true
                          # "350"
                          # "wait for other loop\n to catch up"
                          # "wait till shooter is spun up and feeder is ready\nfor a short while"
                          n176 = local read "Shooter Happy"() -> (w324:bool)
                          n177 = local read "Feeder Happy"() -> (w323:bool)
                          n178 = Wait on Notification(notifier=w319, ignore previous (F)=FALSE) -> (notifier out=w318:refnum<notifier>)  [unwired: 2 in, 3 out]
                          n179 = And(x=w324, y=w323) -> (x .and. y?=w322:bool)
                          n180 = call "CheckShooter.vi"("Time for happy (ms)"=150.0, "Shooter Good?"=w322) -> ("Good to shoot"=w321:bool)  [unwired: 9 in]
                        }
                      }
                      frame #1 {
                        # "wait for other loop\n to catch up"
                        # "shoot the disk!!"
                        n181 = local write "Shoot!"(TRUE ("Shoot!")) -> ()
                        n182 = Wait on Notification(notifier=w327, ignore previous (F)=TRUE) -> (notifier out=w326:refnum<notifier>)  [unwired: 2 in, 3 out]
                      }
                    }
                  }
                }
                frame #3 {
                  # "wait for other loop\n to catch up"
                  # "wait for disk to\nexit shooter"
                  n183 = Wait on Notification(notifier=w330, ignore previous (F)=TRUE) -> (notifier out=w331:refnum<notifier>)  [unwired: 2 in, 3 out]
                  n184 = Wait (ms)(milliseconds to wait=u32 1250) -> ()  [unwired: 1 out]
                }
                frame #4 {
                  # "wait for other loop\n to catch up"
                  # "spin down shooter"
                  n185 = local write "Shooter Speed"(T3."Off" ("Shooter Speed")) -> ()
                  n186 = Wait on Notification(notifier=w335, ignore previous (F)=TRUE) -> (notifier out=w336:refnum<notifier>)  [unwired: 2 in, 3 out]
                }
                frame #5 {
                  # "wait for other loop\n to catch up"
                  # "finish auton mode"
                  n187 = local write "Auton Done"(TRUE ("Auton Done")) -> ()
                  n188 = Wait on Notification(notifier=w338, ignore previous (F)=TRUE) -> ()  [unwired: 2 in, 4 out]
                }
              }
            }
            frame 3 {
              # "MANY shots, back of pyramid --> done"
              n189 = flat-sequence {
                tunnel: [w350] -> w346
                tunnel: w344 -> [w349]
                tunnel: w347 -> [w355]
                tunnel: w346 -> [w353]
                tunnel: [w352] -> w345
                tunnel: w345 -> [w359]
                tunnel: [w358] -> w341
                tunnel: [w380] -> w342
                tunnel: w341 -> [w379]
                tunnel: [w385] -> w343
                tunnel: w342 -> [w384]
                tunnel: w343 -> [w387]
                frame #0 {
                  # "wait for other loop\n to catch up"
                  # "spin up shooter"
                  n190 = local write "Shooter Speed"(T3."Far Pyramid 3pt" ("Shooter Speed")) -> ()
                  n191 = Wait on Notification(notifier=w349, ignore previous (F)=TRUE) -> (notifier out=w350:refnum<notifier>)  [unwired: 2 in, 3 out]
                }
                frame #1 {
                  # "wait for other loop\n to catch up"
                  # "wait [delay] * 1000 ms\nwhich is [delay] seconds"
                  n192 = Multiply(x=w355, y=1000) -> (x*y=w357:u32)
                  n193 = Wait on Notification(notifier=w353, ignore previous (F)=TRUE) -> (notifier out=w352:refnum<notifier>)  [unwired: 2 in, 3 out]
                  n194 = Wait (ms)(milliseconds to wait=w357) -> ()  [unwired: 1 out]
                }
                frame #2 {
                  # "take N shots"
                  n195 = for {
                    N: 25 -> [_]
                    tunnel: w359 -> [w363]
                    tunnel: [w361] -> w358
                    n196 = Cancel Notification(0:w363) -> (8:w364:refnum<notifier>)  [unwired: 1 in, 2 out]
                    n197 = flat-sequence {
                      tunnel: w364 -> [w366]
                      tunnel: [w365] -> w362
                      tunnel: w362 -> [w376]
                      tunnel: [w375] -> w361
                      frame #0 {
                        n198 = while {
                          tunnel: w366 -> [w368]
                          tunnel: [w367] -> w365
                          stop <- w370 stop-if-true
                          # "350"
                          # "wait for other loop\n to catch up"
                          # "wait till shooter is spun up and feeder is ready\nfor a short while"
                          n199 = local read "Shooter Happy"() -> (w373:bool)
                          n200 = local read "Feeder Happy"() -> (w372:bool)
                          n201 = Wait on Notification(notifier=w368, ignore previous (F)=FALSE) -> (notifier out=w367:refnum<notifier>)  [unwired: 2 in, 3 out]
                          n202 = And(x=w373, y=w372) -> (x .and. y?=w371:bool)
                          n203 = call "CheckShooter.vi"("Time for happy (ms)"=150.0, "Shooter Good?"=w371) -> ("Good to shoot"=w370:bool)  [unwired: 9 in]
                        }
                      }
                      frame #1 {
                        # "wait for other loop\n to catch up"
                        # "shoot the disk!!"
                        n204 = local write "Shoot!"(TRUE ("Shoot!")) -> ()
                        n205 = Wait on Notification(notifier=w376, ignore previous (F)=TRUE) -> (notifier out=w375:refnum<notifier>)  [unwired: 2 in, 3 out]
                      }
                    }
                  }
                }
                frame #3 {
                  # "wait for other loop\n to catch up"
                  # "wait for disk to\nexit shooter"
                  n206 = Wait on Notification(notifier=w379, ignore previous (F)=TRUE) -> (notifier out=w380:refnum<notifier>)  [unwired: 2 in, 3 out]
                  n207 = Wait (ms)(milliseconds to wait=u32 1250) -> ()  [unwired: 1 out]
                }
                frame #4 {
                  # "wait for other loop\n to catch up"
                  # "spin down shooter"
                  n208 = local write "Shooter Speed"(T3."Off" ("Shooter Speed")) -> ()
                  n209 = Wait on Notification(notifier=w384, ignore previous (F)=TRUE) -> (notifier out=w385:refnum<notifier>)  [unwired: 2 in, 3 out]
                }
                frame #5 {
                  # "wait for other loop\n to catch up"
                  # "finish auton mode"
                  n210 = local write "Auton Done"(TRUE ("Auton Done")) -> ()
                  n211 = Wait on Notification(notifier=w387, ignore previous (F)=TRUE) -> ()  [unwired: 2 in, 4 out]
                }
              }
            }
          }
        }
        frame 3 {
          n212 = case shown="1" w393 {
            tunnel: w392 -> [_ w423]
            tunnel: w391 -> [_ w426]
            tunnel: w390 -> [_ w415]
            frame 0, Default {
              # "do nothing"
            }
            frame 1 {
              # "WORK IN PROGRESS"
              # "MANY shots, back RIGHT of pyramid --> pickup close 2 --> shoot 2 --> done"
              n213 = flat-sequence {
                tunnel: [w429] -> w425
                tunnel: w423 -> [w428]
                tunnel: w426 -> [w434]
                tunnel: w425 -> [w432]
                tunnel: [w431] -> w424
                tunnel: w424 -> [w438]
                tunnel: [w437] -> w421
                tunnel: [w459] -> w420
                tunnel: w421 -> [w458]
                tunnel: w420 -> [w462]
                tunnel: [w463] -> w419
                tunnel: [w471] -> w418
                tunnel: w419 -> [w470]
                tunnel: w415 -> [w469]
                tunnel: [w467] -> w414
                tunnel: w418 -> [w478]
                tunnel: [w479] -> w416
                tunnel: w414 -> [w477]
                tunnel: [w476] -> w413
                tunnel: [w485] -> w417
                tunnel: w416 -> [w484]
                tunnel: w413 -> [w482]
                tunnel: [w481] -> w412
                tunnel: [w496] -> w397
                tunnel: w417 -> [w495]
                tunnel: w412 -> [w492]
                tunnel: [w491] -> w395
                tunnel: w397 -> [w504]
                tunnel: [w503] -> w396
                tunnel: w395 -> [w500]
                tunnel: [w499] -> w394
                tunnel: w396 -> [w511]
                tunnel: [w512] -> w399
                tunnel: [w507] -> w398
                tunnel: w394 -> [w508]
                tunnel: [w519] -> w409
                tunnel: w399 -> [w518]
                tunnel: w398 -> [w516]
                tunnel: [w515] -> w408
                tunnel: [w514] -> w407
                tunnel: w409 -> [w526]
                tunnel: [w527] -> w406
                tunnel: w408 -> [w529]
                tunnel: [w529] -> w404
                tunnel: w407 -> [w523]
                tunnel: [w521] -> w402
                tunnel: w406 -> [w532]
                tunnel: [w533] -> w405
                tunnel: w404 -> [w535]
                tunnel: [w535] -> w403
                tunnel: w402 -> [w530]
                tunnel: [w539] -> w401
                tunnel: w405 -> [w538]
                tunnel: w403 -> [w537]
                tunnel: w401 -> [w550]
                tunnel: [w551] -> w400
                tunnel: [w554] -> w411
                tunnel: w400 -> [w553]
                tunnel: w411 -> [w575]
                tunnel: [w576] -> w410
                tunnel: [w580] -> w422
                tunnel: w410 -> [w579]
                tunnel: w422 -> [w582]
                frame #0 {
                  # "wait for other loop\n to catch up"
                  # "spin up shooter"
                  n214 = local write "Shooter Speed"(T3."Far Pyramid 3pt" ("Shooter Speed")) -> ()
                  n215 = Wait on Notification(notifier=w428, ignore previous (F)=TRUE) -> (notifier out=w429:refnum<notifier>)  [unwired: 2 in, 3 out]
                }
                frame #1 {
                  # "wait for other loop\n to catch up"
                  # "wait [delay] * 1000 ms\nwhich is [delay] seconds"
                  n216 = Multiply(x=w434, y=1000) -> (x*y=w436:u32)
                  n217 = Wait on Notification(notifier=w432, ignore previous (F)=TRUE) -> (notifier out=w431:refnum<notifier>)  [unwired: 2 in, 3 out]
                  n218 = Wait (ms)(milliseconds to wait=w436) -> ()  [unwired: 1 out]
                }
                frame #2 {
                  # "take N shots"
                  n219 = for {
                    N: 5 -> [_]
                    tunnel: w438 -> [w442]
                    tunnel: [w440] -> w437
                    n220 = Cancel Notification(0:w442) -> (8:w443:refnum<notifier>)  [unwired: 1 in, 2 out]
                    n221 = flat-sequence {
                      tunnel: w443 -> [w445]
                      tunnel: [w444] -> w441
                      tunnel: w441 -> [w455]
                      tunnel: [w454] -> w440
                      frame #0 {
                        n222 = while {
                          tunnel: w445 -> [w447]
                          tunnel: [w446] -> w444
                          stop <- w449 stop-if-true
                          # "wait for other loop\n to catch up"
                          # "wait till shooter is spun up and feeder is ready\nfor a short while"
                          n223 = local read "Shooter Happy"() -> (w452:bool)
                          n224 = local read "Feeder Happy"() -> (w451:bool)
                          n225 = Wait on Notification(notifier=w447, ignore previous (F)=FALSE) -> (notifier out=w446:refnum<notifier>)  [unwired: 2 in, 3 out]
                          n226 = And(x=w452, y=w451) -> (x .and. y?=w450:bool)
                          n227 = call "CheckShooter.vi"("Time for happy (ms)"=350.0, "Shooter Good?"=w450) -> ("Good to shoot"=w449:bool)  [unwired: 9 in]
                        }
                      }
                      frame #1 {
                        # "wait for other loop\n to catch up"
                        # "shoot the disk!!"
                        n228 = local write "Shoot!"(TRUE ("Shoot!")) -> ()
                        n229 = Wait on Notification(notifier=w455, ignore previous (F)=TRUE) -> (notifier out=w454:refnum<notifier>)  [unwired: 2 in, 3 out]
                      }
                    }
                  }
                }
                frame #3 {
                  # "wait for other loop\n to catch up"
                  # "wait for disk to\nexit shooter"
                  n230 = Wait on Notification(notifier=w458, ignore previous (F)=TRUE) -> (notifier out=w459:refnum<notifier>)  [unwired: 2 in, 3 out]
                  n231 = Wait (ms)(milliseconds to wait=u32 400) -> ()  [unwired: 1 out]
                }
                frame #4 {
                  # "wait for other loop\n to catch up"
                  # "set up for driving"
                  n232 = local write "Stop Drive"(FALSE ("Shift Low")) -> ()
                  n233 = local write "Shift Low"(TRUE ("Shift Low")) -> ()
                  n234 = Wait on Notification(notifier=w462, ignore previous (F)=TRUE) -> (notifier out=w463:refnum<notifier>)  [unwired: 2 in, 3 out]
                }
                frame #5 {
                  # "turn to faceaway\nfrom  goals\nstart at right side"
                  # "wait for other loop\n to catch up"
                  n235 = call "AutoTurnGyro.vi"("Turn Amount"=-30, "Initial Angle"=w469) -> ("Target Angle Out"=w467:dbl)  [unwired: 8 in, 1 out]
                  n236 = Wait on Notification(notifier=w470, ignore previous (F)=TRUE) -> (notifier out=w471:refnum<notifier>)  [unwired: 2 in, 3 out]
                }
                frame #6 {
                  # "wait for other loop\n to catch up"
                  # "drive backwars"
                  n237 = Wait on Notification(notifier=w478, ignore previous (F)=TRUE) -> (notifier out=w479:refnum<notifier>)  [unwired: 2 in, 3 out]
                  n238 = call "AutoDistanceGyro.vi"("InitialAngle"=w477, "Reset Encoders"=TRUE, "TargetDistance"=-54.0, "Motor Speed"=-0.6) -> ("InitialAngle Out"=w476:dbl)  [unwired: 10 in, 1 out]
                }
                frame #7 {
                  # "wait for other loop\n to catch up"
                  # "turn to face disks\nand start DAD and DT"
                  n239 = Wait on Notification(notifier=w484, ignore previous (F)=TRUE) -> (notifier out=w485:refnum<notifier>)  [unwired: 2 in, 3 out]
                  n240 = call "AutoTurnGyro.vi"("Turn Amount"=-90, "Initial Angle"=w482) -> ("Target Angle Out"=w481:dbl)  [unwired: 8 in, 1 out]
                }
                frame #8 {
                  # "wait for other loop\n to catch up"
                  # "start to drive over disks"
                  n241 = Wait on Notification(notifier=w495, ignore previous (F)=TRUE) -> (notifier out=w496:refnum<notifier>)  [unwired: 2 in, 3 out]
                  n242 = local write "DAD Output"(WPI_RelayValue."On" ("DAD Output")) -> ()
                  n243 = call "AutoDistanceGyro.vi"("InitialAngle"=w492, "Reset Encoders"=TRUE, "TargetDistance"=20.0, "Motor Speed"=0.6) -> ("InitialAngle Out"=w491:dbl)  [unwired: 10 in, 1 out]
                  n244 = local write "DT Output"(enum16{"Off", "Up", "Down"}."Up" ("DT Output")) -> ()
                  n245 = local write "DAD Up"(FALSE ("DAD Up")) -> ()
                }
                frame #9 {
                  # "after under pyramid\npop up shooter"
                  # "wait for other loop\n to catch up"
                  n246 = local write "Shooter Up"(TRUE ("DAD Up")) -> ()
                  n247 = Wait on Notification(notifier=w504, ignore previous (F)=TRUE) -> (notifier out=w503:refnum<notifier>)  [unwired: 2 in, 3 out]
                  n248 = call "AutoDistanceGyro.vi"("InitialAngle"=w500, "TargetDistance"=40.0, "Motor Speed"=0.6) -> ("InitialAngle Out"=w499:dbl)  [unwired: 11 in, 1 out]
                }
                frame #10 {
                  # "wait for pop up then\npop down"
                  # "wait for other loop\n to catch up"
                  n249 = local write "Shooter Up"(FALSE ("DAD Up")) -> ()
                  n250 = Wait on Notification(notifier=w511, ignore previous (F)=TRUE) -> (notifier out=w512:refnum<notifier>)  [unwired: 2 in, 3 out]
                  n251 = call "AutoDistanceGyro.vi"("InitialAngle"=w508, "TargetDistance"=112.0, "Motor Speed"=0.6) -> ("InitialAngle Out"=w507:dbl)  [unwired: 11 in, 1 out]
                }
                frame #11 {
                  # "wait for other loop\n to catch up"
                  # "turn to goals\nstart counting for\nDT slowness"
                  n252 = Wait on Notification(notifier=w518, ignore previous (F)=TRUE) -> (notifier out=w519:refnum<notifier>)  [unwired: 2 in, 3 out]
                  n253 = Tick Count (ms)() -> (millisecond timer value=w515:u32)
                  n254 = call "AutoTurnGyro.vi"("Turn Amount"=90, "Initial Angle"=w516) -> ("Target Angle Out"=w514:dbl)  [unwired: 8 in, 1 out]
                }
                frame #12 {
                  # "wait for other loop\n to catch up"
                  # "drive to close\npyramid"
                  n255 = Wait on Notification(notifier=w526, ignore previous (F)=TRUE) -> (notifier out=w527:refnum<notifier>)  [unwired: 2 in, 3 out]
                  n256 = call "AutoDistanceGyro.vi"("InitialAngle"=w523, "Reset Encoders"=TRUE, "TargetDistance"=54.0, "Motor Speed"=0.6) -> ("InitialAngle Out"=w521:dbl)  [unwired: 10 in, 1 out]
                }
                frame #13 {
                  # "aim at goals"
                  # "wait for other loop\n to catch up"
                  n257 = Wait on Notification(notifier=w532, ignore previous (F)=TRUE) -> (notifier out=w533:refnum<notifier>)  [unwired: 2 in, 3 out]
                  n258 = call "AutoTurnGyro.vi"("Turn Amount"=-60, "Initial Angle"=w530) -> ()  [unwired: 8 in, 2 out]
                }
                frame #14 {
                  # "wait for other loop\n to catch up"
                  # "make sure DT has caught up\nand finsih driving"
                  n259 = while {
                    tunnel: w537 -> [w543]
                    stop <- w546 stop-if-true
                    # "wait for 10 ms every\nloop not to hog resources"
                    n260 = Wait (ms)(milliseconds to wait=10) -> (millisecond timer value=w541:u32)
                    n261 = Add(x=w543, y=7000) -> (x+y=w542:u32)
                    n262 = Greater?(x=w541, y=w542) -> (0:w546:bool)
                  }
                  n263 = local write "Stop Drive"(TRUE ("Shift Low")) -> ()
                  n264 = Wait on Notification(notifier=w538, ignore previous (F)=TRUE) -> (notifier out=w539:refnum<notifier>)  [unwired: 2 in, 3 out]
                }
                frame #15 {
                  # "wait for other loop\n to catch up"
                  # "spend a split\nseccond turning\nstuff off"
                  n265 = local write "DAD Output"(WPI_RelayValue."Off" ("DAD Output")) -> ()
                  n266 = local write "DT Output"(enum16{"Off", "Up", "Down"}."Off" ("DT Output")) -> ()
                  n267 = local write "DAD Up"(TRUE ("DAD Up")) -> ()
                  n268 = Wait on Notification(notifier=w550, ignore previous (F)=TRUE) -> (notifier out=w551:refnum<notifier>)  [unwired: 2 in, 3 out]
                }
                frame #16 {
                  # "take N shots"
                  # "Shoot disks"
                  n269 = for {
                    N: 8 -> [_]
                    tunnel: w553 -> [w558]
                    tunnel: [w556] -> w554
                    n270 = Cancel Notification(0:w558) -> (8:w559:refnum<notifier>)  [unwired: 1 in, 2 out]
                    n271 = flat-sequence {
                      tunnel: w559 -> [w561]
                      tunnel: [w560] -> w557
                      tunnel: w557 -> [w571]
                      tunnel: [w570] -> w556
                      frame #0 {
                        n272 = while {
                          tunnel: w561 -> [w563]
                          tunnel: [w562] -> w560
                          stop <- w565 stop-if-true
                          # "wait for other loop\n to catch up"
                          # "wait till shooter is spun up and feeder is ready\nfor a short while"
                          n273 = local read "Shooter Happy"() -> (w568:bool)
                          n274 = local read "Feeder Happy"() -> (w567:bool)
                          n275 = Wait on Notification(notifier=w563, ignore previous (F)=FALSE) -> (notifier out=w562:refnum<notifier>)  [unwired: 2 in, 3 out]
                          n276 = And(x=w568, y=w567) -> (x .and. y?=w566:bool)
                          n277 = call "CheckShooter.vi"("Time for happy (ms)"=350.0, "Shooter Good?"=w566) -> ("Good to shoot"=w565:bool)  [unwired: 9 in]
                        }
                      }
                      frame #1 {
                        # "wait for other loop\n to catch up"
                        # "shoot the disk!!"
                        n278 = local write "Shoot!"(TRUE ("Shoot!")) -> ()
                        n279 = Wait on Notification(notifier=w571, ignore previous (F)=TRUE) -> (notifier out=w570:refnum<notifier>)  [unwired: 2 in, 3 out]
                      }
                    }
                  }
                }
                frame #17 {
                  # "make sure disks\nexist shooter"
                  # "wait for other loop\n to catch up"
                  n280 = Wait on Notification(notifier=w575, ignore previous (F)=TRUE) -> (notifier out=w576:refnum<notifier>)  [unwired: 2 in, 3 out]
                  n281 = Wait (ms)(milliseconds to wait=u32 750) -> ()  [unwired: 1 out]
                }
                frame #18 {
                  # "wait for other loop\n to catch up"
                  # "spin down shooter"
                  n282 = local write "Shooter Speed"(T3."Off" ("Shooter Speed")) -> ()
                  n283 = Wait on Notification(notifier=w579, ignore previous (F)=TRUE) -> (notifier out=w580:refnum<notifier>)  [unwired: 2 in, 3 out]
                }
                frame #19 {
                  # "wait for other loop\n to catch up"
                  # "finish auton mode"
                  n284 = local write "Auton Done"(TRUE ("Auton Done")) -> ()
                  n285 = Wait on Notification(notifier=w582, ignore previous (F)=TRUE) -> ()  [unwired: 2 in, 4 out]
                }
              }
            }
          }
        }
      }
    }
  }
